vi "Get External Xp.vi"(8 "error in":errorcluster, 11 "VISA resource name in":refnum<visa-resource-name>) -> (0 "error out":errorcluster, 1 "ExternalXp (out)":dbl, 3 "VISA resource name out":refnum<visa-resource-name>)   [LabVIEW 2018, in "JULABO DeviceDriver.lvlib"]
doc: "This VI returns the Proportional component <B>Xp</B> in case of external temperature control.\n\nNote:\nThis function is not available for devices which do not have an external sensor plug."
uses:
  JULABO DeviceDriver.lvlib
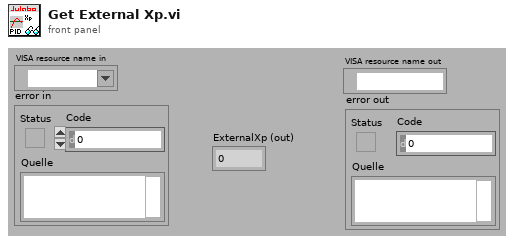
[diagram p1: front panel]
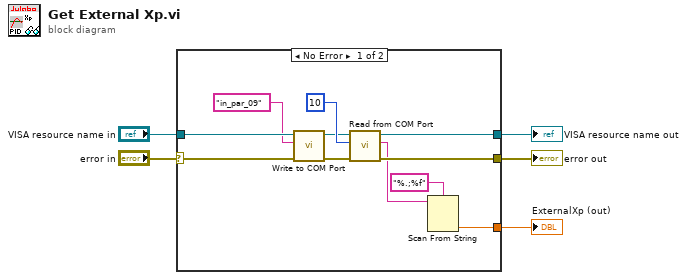
[diagram p0: block diagram]
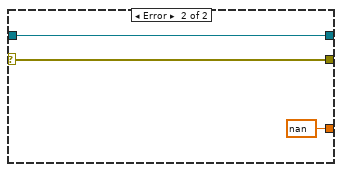
[diagram p2: hidden frame]
diagram:
  n1 = case shown="No Error" "error in" {
    selector: "error in" -> [w13 w18]
    tunnel: [w16 w19] -> w5
    tunnel: [w15 w18] -> w4
    tunnel: "VISA resource name in" -> [w14 w19]
    tunnel: [w6 nan] -> w1
    frame No Error {
      n2 = call "Write to COM Port.vi"("error in"=w13, "Command (input)"="in_par_09" ("Schreibpuffer"), "VISA resource name in"=w14) -> ("error out"=w8:errorcluster, "VISA resource name out"=w9:refnum<visa-resource-name>)  [unwired: 7 in]
      n3 = call "Read from COM Port.vi"("error in"=w8, "Byte to Read (-1:All)"=u32 10 ("Anzahl der Byte"), "VISA resource name in"=w9) -> ("error out"=w15:errorcluster, "String (output)"=w11:string, "VISA resource name out"=w16:refnum<visa-resource-name>)  [unwired: 5 in, 1 out]
      n4 = Scan From String(format string="%.;%f" ("Format-String"), input string=w11) -> (output 1=w6:dbl)  [unwired: 3 in, 3 out]
    }
    frame Error {
    }
  }
  "VISA resource name out" <- w5
  "error out" <- w4
  "ExternalXp (out)" <- w1
